vi "resetOutput.vi"(8 "error in (no error)":errorcluster, 11 "DIO64Output in":refnum<class "DIO64Output.lvclass">) -> (0 "error out":errorcluster, 3 "DIO64Output out":refnum<class "DIO64Output.lvclass">)   [LabVIEW 2011, in "Hardware.lvlib" / "Channels.lvlib" / "DIO64Output.lvclass"]
uses:
  DIO64Output.lvclass
  <userlib>/dio64_32.LLB/DIO64 Out Config Control.ctl
  <userlib>/dio64_32.LLB/DIO64 clock control.ctl
  <userlib>/dio64_32.LLB/DIO64 start trig.ctl
  <userlib>/dio64_32.LLB/DIO64 stop trig.ctl
  DIO64Output.lvclass/DIO64Output.ctl
  DigitalOutput.lvclass
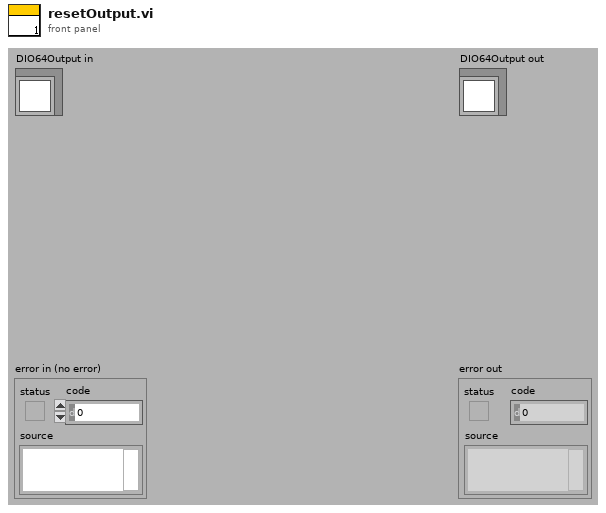
[diagram p1: front panel]
types:
  T1 = typedef "DIO64 Out Config Control.ctl" = cluster{"flags":enum16{"unused"}, "clock control":T2, "start trigger":T3, "stop trigger":T4, "DAQ clock modulo":u32, "repetitions":u32, "#transitions":u16}
  T2 = typedef "DIO64 clock control.ctl" = enum16{"internal", "external", "trig 0", "OCXO"}
  T3 = typedef "DIO64 start trig.ctl" = cluster{"source":enum16{"none", "internal", "external", "trig 2", "PXI Star"}, "type":enum16{"level", "edge", "edge to edge"}, "sense":enum16{"rising", "falling"}}
  T4 = typedef "DIO64 stop trig.ctl" = cluster{"source":enum16{"none", "internal", "external", "trig 3 in", "output FIFO"}, "type":enum16{"level", "edge"}, "sense":enum16{"falling", "rising"}}
  T5 = typedef "DIO64 Out Status.ctl" = cluster{"pktsize":u16, "portCount":u16, "writePtr":u16, "readPtr":u16, "time0":u16, "time1":u16, "fifoSize":u32, "fifo0":u16, "ticks":u32, "flags":u16, "clkControl":u16, "startControl":u16, "stopControl":u16, "AIControl":u32, "AICurrent":u16, "startTime0":u16, "startTime1":u16, "stopTime0":u16, "stopTime1":u16, "cur trans":u32, "cur reps":u32}
  T6 = cluster{"Timestamps ms":dbl[], "DataPerChannel":dbl[][]}
  T7 = cluster{"Timestamps ms":dbl[], "Bitmap":bool[][]}
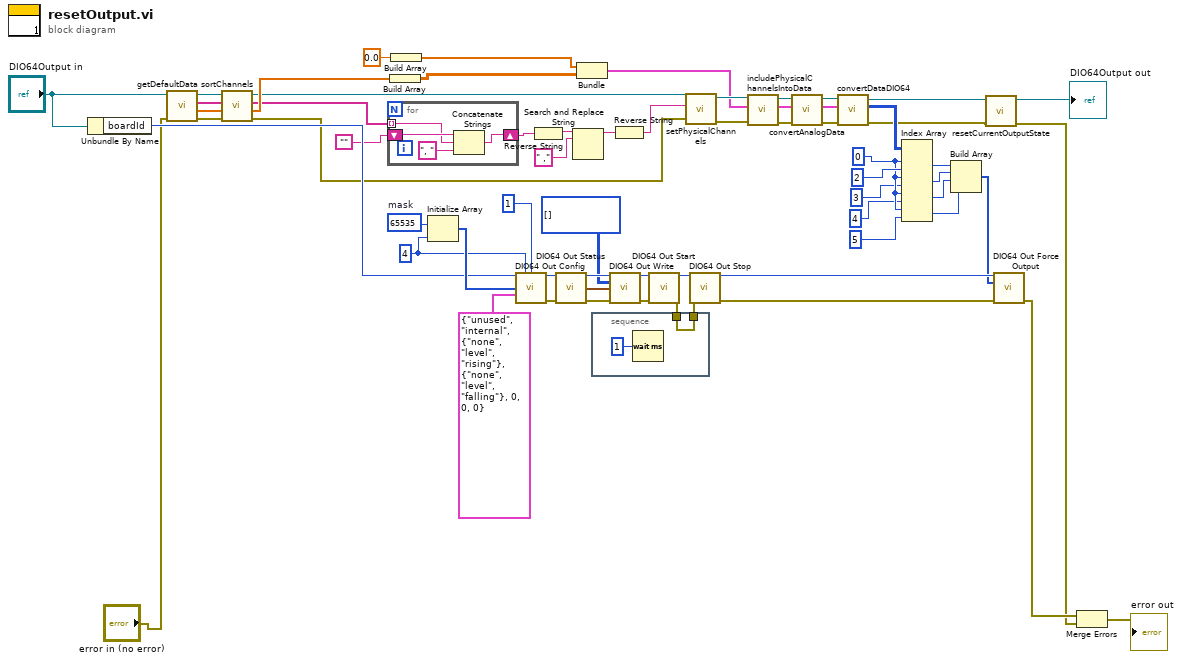
[diagram p0: block diagram]
diagram:
  w17 = 0
  w55 = 4
  w54 = u16 65535  # mask
  n1 = Unbundle By Name("DIO64Output in") -> ("boardId"=w46:i32)
  n2 = call "getDefaultData.vi"("error in (no error)"="error in (no error)", "DigitalOutput in"="DIO64Output in") -> ("error out"=w8:errorcluster, "calibratedValues"=w6:dbl[], "channel_addresses"=w4:string[], "DigitalOutput out"=w2:refnum<class "DIO64Output.lvclass">)  [unwired: 6 in]
  n3 = call "sortChannels.vi"("error in (no error)"=w8, "calibratedValues"=w6, "channel_addresses"=w4, "DIO64Output in"=w2) -> ("error out"=w7:errorcluster, "sorted Data"=w5:dbl[], "sorted channels addresses"=w3:string[], "DIO64Output out"=w1:refnum<class "DIO64Output.lvclass">)  [unwired: 4 in]
  n4 = for {
    tunnel: w3 -> [w67] mode=indexing
    shift-right: [w65] -> w39
    shift-left: "" -> [w68]
    n5 = Concatenate Strings(w68, w67, ", ") -> (w65:string)
  }
  n6 = Build Array(w5) -> (w31:dbl[][])
  n7 = Build Array(0.0) -> (w32:dbl[])
  n8 = Initialize Array(w54, w55) -> (w56:u16[])
  n9 = call <userlib>:"DIO64 Out Config.vi"("board in"=w46, "#ports"=w55, "divider"=u32 1, "mask"=w56, "Config Control"=T1 {"flags"=enum."unused", "clock control"=enum."internal", "start trigger"={"source"=enum."none", "type"=enum."level", "sense"=enum."rising"}, "stop trigger"={"source"=enum."none", "type"=enum."level", "sense"=enum."falling"}, "DAQ clock modulo"=0, "repetitions"=0, "#transitions"=0}) -> ("board out"=w63:u16, "error out"=w64:errorcluster)  [unwired: 8 in, 1 out]
  n10 = Reverse String(1:w39) -> (0:w38:string)
  n11 = call <userlib>:"DIO64 Out Status.vi"("board in"=w63, "error in (no error)"=w64) -> ("board out"=w60:u16, "Out Status"=w59:T5, "error out"=w57:errorcluster)  [unwired: 10 in, 1 out]
  n12 = Search and Replace String(input string=w38, search string=" ,") -> (result string=w36:string)  [unwired: 6 in, 3 out]
  n13 = Bundle(w32, w31) -> (w30:cluster{dbl[], dbl[][]})  [unwired: 1 in]
  n14 = call <userlib>:"DIO64 Out Write.vi"("board in"=w60, "data"=u16[][] [] ("Timestamp and Data Array for each board"), "Out Status"=w59, "error in (no error)"=w57) -> ("board out"=w61:u16, "error out"=w58:errorcluster)  [unwired: 10 in]
  n15 = Reverse String(1:w36) -> (0:w35:string)
  n16 = call <userlib>:"DIO64 Out Start.vi"("board in"=w61, "error in (no error)"=w58) -> ("board out"=w62:u16, "error out"=w51:errorcluster)  [unwired: 12 in]
  n17 = stacked-sequence {
    tunnel: w51 -> [w70]
    tunnel: [w70] -> w50
    frame #0 {
      n18 = Wait (ms)(milliseconds to wait=u32 1) -> ()  [unwired: 1 out]
    }
  }
  n19 = call-dynamic "setPhysicalChannels.vi"("error in (no error)"=w7, "Physical Channels"=w35, "DigitalOutput.lvclass in"=w1) -> ("error out"=w33:errorcluster, "DigitalOutput.lvclass out"=w34:refnum<class "DIO64Output.lvclass">)  [unwired: 7 in]
  n20 = call <userlib>:"DIO64 Out Stop.vi"("board in"=w62, "error in (no error)"=w50) -> ("board out"=w47:u16, "error out"=w48:errorcluster)  [unwired: 12 in]
  n21 = call "includePhysicalChannelsIntoData.vi"("error in (no error)"=w33, "Data"=w30, "DIO64Output in"=w34) -> ("error out"=w29:errorcluster, "Data out"=w27:T6, "DIO64Output out"=w28:refnum<class "DIO64Output.lvclass">)  [unwired: 6 in]
  n22 = call "convertAnalogData.vi"("error in (no error)"=w29, "Data"=w27, "DIO64Output in"=w28) -> ("error out"=w25:errorcluster, "digitalData"=w26:T7, "DIO64Output out"=w24:refnum<class "DIO64Output.lvclass">)  [unwired: 6 in]
  n23 = call "convertDataDIO64.vi"("error in (no error)"=w25, "Data"=w26, "DIO64Output in"=w24) -> ("error out"=w20:errorcluster, "data"=w23:u16[][], "DIO64Output out"=w22:refnum<class "DIO64Output.lvclass">)  [unwired: 4 in, 2 out]
  n24 = Index Array(array=w23, index (row) #1=w17, index (col) #1=2, index (row) #2=w17, index (col) #2=3, index (row) #3=w17, index (col) #3=4, index (row) #4=w17, index (col) #4=5) -> (element #1=w13:u16, element #2=w12:u16, element #3=w10:u16, element #4=w11:u16)
  n25 = Build Array(w13, w12, w10, w11) -> (w9:u16[])
  n26 = call "resetCurrentOutputState.vi"("error in (no error)"=w20, "DigitalOutput in"=w22) -> ("error out"=w19:errorcluster, "DigitalOutput out"=→"DIO64Output out":refnum<class "DIO64Output.lvclass">)  [unwired: 8 in]
  n27 = call <userlib>:"DIO64 Out Force Output.vi"("board in"=w47, "data"=w9, "error in (no error)"=w48) -> ("error out"=w45:errorcluster)  [unwired: 11 in, 1 out]
  n28 = Merge Errors(w45, w19) -> (→"error out":errorcluster)
